vi "Write Multiple Holding Registers.vi"(8 "error in":errorcluster, 9 "registers to write":u16[](array[numeric]), 10 "starting address":u16, 11 "Modbus master in":refnum<class "Modbus Master.lvclass">) -> (0 "error out":errorcluster, 3 "Modbus master out":refnum<class "Modbus Master.lvclass">)   [LabVIEW 2012, in "Modbus Master.lvclass"]
doc: "Writes <B>registers to write</B> starting at <B>starting address</B> to the device holding registers."
uses:
  Modbus Master.lvclass
  Modbus API.lvclass/Modbus API.ctl
  Modbus Master.lvclass/Modbus Master.ctl
  Transmission Data Unit/Transmission Data Unit.lvclass
  Master Function Definition/Master Function Definition.lvclass
  Modbus API.lvclass
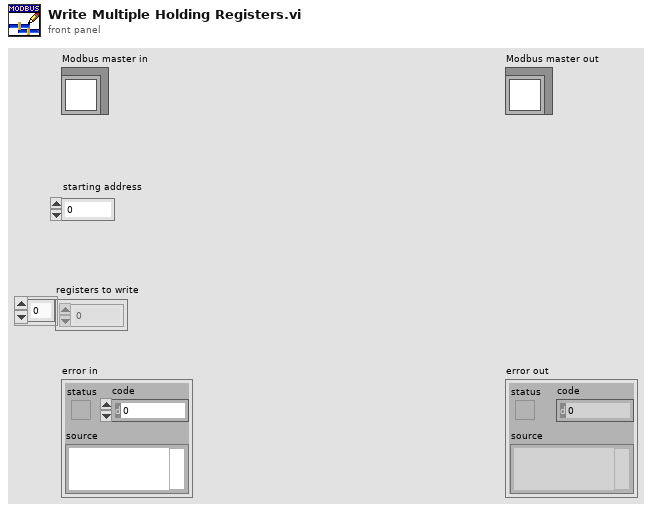
[diagram p1: front panel]
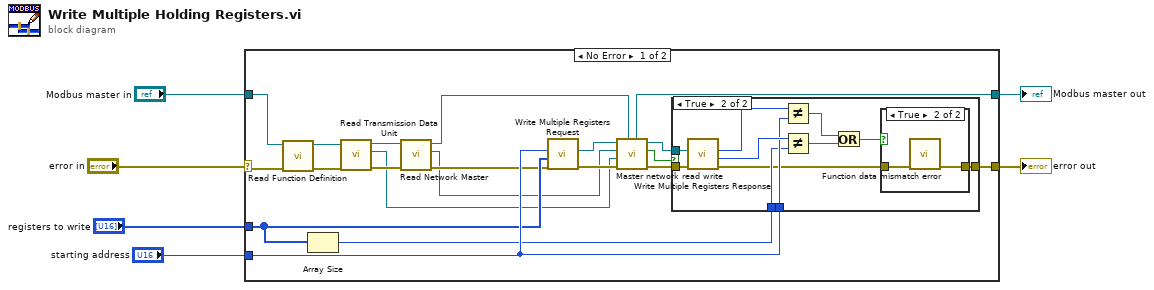
[diagram p0: block diagram]
diagram:
  n1 = case shown="No Error" "error in" {
    selector: "error in" -> [w14 w43]
    tunnel: "Modbus master in" -> [w13 w42]
    tunnel: [w25 w43] -> w3
    tunnel: [w18 w42] -> w4
    tunnel: "registers to write" -> [w22 _]
    tunnel: "starting address" -> [w24 _]
    frame No Error {
      n2 = call "Read Function Definition.vi"("error in"=w14, "Modbus master in"=w13) -> ("error out"=w15:errorcluster, "Modbus master out"=w12:refnum<class "Modbus Master.lvclass">)  [unwired: 7 in, 1 out]
      n3 = Array Size(array=w22) -> (size(s)=w23:i32)
      n4 = call "Read Transmission Data Unit.vi"("error in"=w15, "Modbus instance in"=w12) -> ("error out"=w17:errorcluster, "transmission data unit"=w8:refnum<class "Transmission Data Unit.lvclass">, "Modbus instance out"=w11:refnum<class "Modbus Master.lvclass">)  [unwired: 7 in]
      n5 = call "Read Network Master.vi"("error in"=w17, "Modbus master in"=w11) -> ("error out"=w16:errorcluster, "network master"=w9:refnum<class "Network Master.lvclass">, "Modbus master out"=w10:refnum<class "Modbus Master.lvclass">)  [unwired: 7 in]
      n6 = call "Write Multiple Registers Request.vi"("error in"=w16, "Registers"=w22, "Starting Address"=w24) -> ("error out"=w26:errorcluster, "modbus data unit out"=w20:refnum<class "Modbus Data Unit.lvclass">)  [unwired: 7 in]
      n7 = call "Master network read write.vi"("Modbus master in"=w10, "error in"=w26, "transmission data unit in"=w8, "network master in"=w9, "Modbus data unit in"=w20) -> ("error out"=w21:errorcluster, "PDU Valid?"=w7:bool, "Modbus data unit out"=w19:refnum<class "Modbus Data Unit.lvclass">, "Modbus master out"=w18:refnum<class "Modbus Master.lvclass">)  [unwired: 3 in]
      n8 = case shown="True" w7 {
        tunnel: [w27 w35] -> w25
        tunnel: w24 -> [_ w32]
        tunnel: w23 -> [_ w31]
        tunnel: w21 -> [w27 w30]
        tunnel: w19 -> [_ w29]
        frame False {
        }
        frame True {
          n9 = call "Write Multiple Registers Response.vi"("error in"=w30, "modbus data unit in"=w29) -> ("error out"=w28:errorcluster, "Number of Registers"=w33:u16, "Start Address"=w34:u16)  [unwired: 7 in]
          n10 = Not Equal?(x=w34, y=w32) -> (x != y?=w37:bool)
          n11 = Not Equal?(x=w33, y=w31) -> (x != y?=w36:bool)
          n12 = Or(x=w37, y=w36) -> (x .or. y?=w38:bool)
          n13 = case shown="True" w38 {
            tunnel: [w39 w41] -> w35
            tunnel: w28 -> [w39 w40]
            frame False {
            }
            frame True {
              n14 = call "Function data mismatch error.vi"("error in (no error)"=w40) -> ("error out"=w41:errorcluster)  [unwired: 10 in]
            }
          }
        }
      }
    }
    frame Error {
    }
  }
  "error out" <- w3
  "Modbus master out" <- w4
